vi "State Mechine.vi"() -> ()   [LabVIEW 2015]
uses:
  Control 2.ctl
  Control 3.ctl
panel:
  out "Sine":dynamicdata(graph)
  in  "STOP/START":bool
  out "STATE":string="START"
  out "Vertical Fill Slide 2":T1 scale=0.0..10.0
  in  "Vertical Fill Slide":T1 scale=0.0..10.0
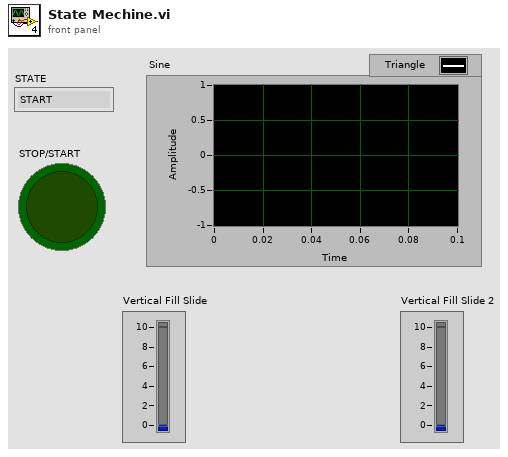
[diagram p1: front panel]
types:
  T1 = typedef "Control 2.ctl" = dbl
  T2 = typedef "Control 3.ctl" = enum16{"START", "INITIALIZE", "PROCCES1", "PROCCES2", "PROCCES3", "CONTINUED?", "STOP"}
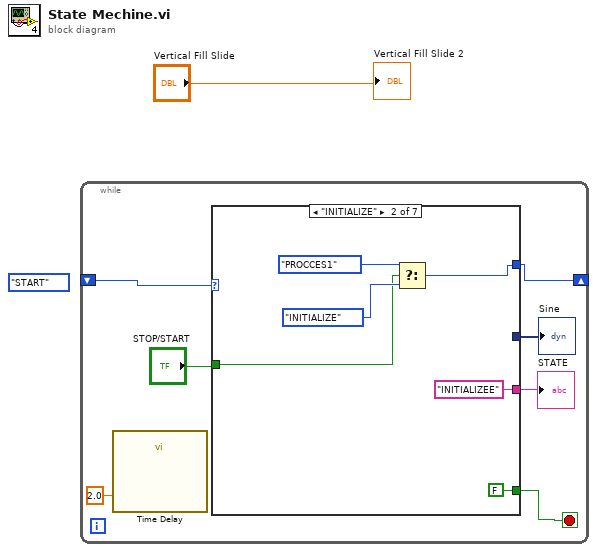
[diagram p0: block diagram]
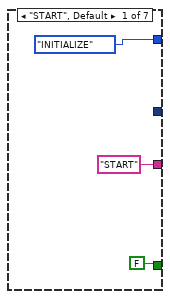
[diagram p2: hidden frame]
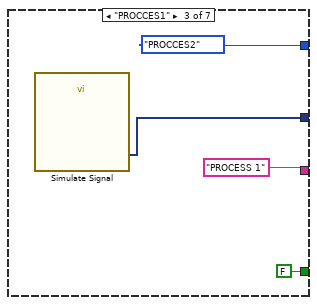
[diagram p3: hidden frame]
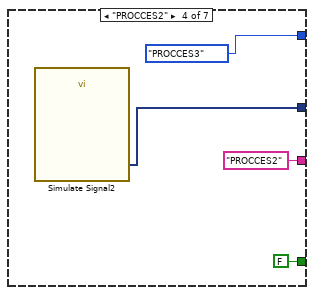
[diagram p4: hidden frame]
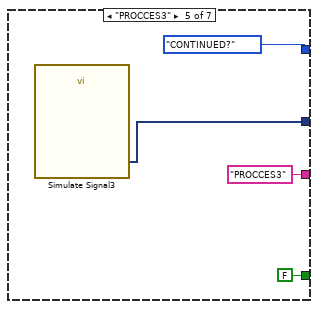
[diagram p5: hidden frame]
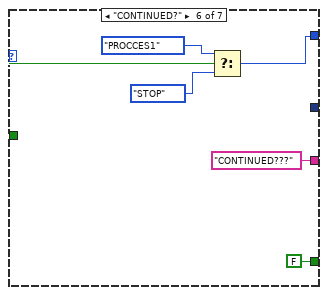
[diagram p6: hidden frame]
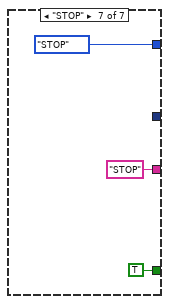
[diagram p7: hidden frame]
diagram:
  (unwired) Control_3."START"
  n1 = while {
    shift-right: [w7] -> _
    shift-left: _ -> [w8]
    stop <- w6 stop-if-true
    n2 = call "Time Delay"("Delay Time (s)"=2.0) -> ()  [unwired: 10 in, 1 out]
    n3 = case shown="\"INITIALIZE\"" w8 {
      tunnel: [Control_3."INITIALIZE" w15 Control_3."PROCCES2" Control_3."PROCCES3" Control_3."CONTINUED?" w32 Control_3."STOP"] -> w7
      tunnel: [FALSE FALSE FALSE FALSE FALSE FALSE TRUE] -> w6
      tunnel: ["START" "INITIALIZEE" "PROCESS 1" "PROCCES2" "PROCCES3" "CONTINUED???" "STOP"] -> w5
      tunnel: "STOP/START" -> [_ w12 _ _ _ w34 _]
      tunnel: [_ _ w19 w22 w26 _ _] -> w3
      frame "START", Default {
      }
      frame "INITIALIZE" {
        n4 = Select(t=Control_3."PROCCES1", s=w12, f=Control_3."INITIALIZE") -> (s? t:f=w15:T2)
      }
      frame "PROCCES1" {
        n5 = call "Simulate Signal"() -> ("Sine"=w19:dynamicdata)  [unwired: 14 in, 1 out]
      }
      frame "PROCCES2" {
        n6 = call "Simulate Signal2"() -> ("Triangle"=w22:dynamicdata)  [unwired: 14 in, 1 out]
      }
      frame "PROCCES3" {
        n7 = call "Simulate Signal3"() -> ("Sawtooth"=w26:dynamicdata)  [unwired: 14 in, 1 out]
      }
      frame "CONTINUED?" {
        n8 = Select(t=Control_3."PROCCES1", s=w34, f=Control_3."STOP") -> (s? t:f=w32:T2)
      }
      frame "STOP" {
      }
    }
    "STATE" <- w5
    "Sine" <- w3
  }
  "Vertical Fill Slide 2" <- "Vertical Fill Slide"
